vi "parse_int8.vi"   [LabVIEW 2016]
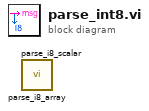
[diagram p0: block diagram]
diagram:
  n1 = call "parse_i8_array.vi"() -> ()  [unwired: 5 in, 3 out]
  n2 = call "parse_i8_scalar.vi"() -> ()  [unwired: 5 in, 3 out]
